vi "Send Current.vi"(8 "error in":errorcluster, 11 "6700C in":refnum<class "6700C.lvclass">) -> (0 "error out":errorcluster, 3 "6700C out":refnum<class "6700C.lvclass">)   [LabVIEW 2019, in "6700C.lvlib" / "6700C.lvclass"]
uses:
  Library/6700C.lvclass
  C:/Users/Public/Documents/Development/builds/Instruments/PowerSupply.lvlibp/Library/PowerSupply.lvclass
  Library/6700C.lvclass/6700C.ctl
  Accessors/Read Local Resource.vi
  Accessors/Write Local Resource.vi
  builds/Instruments/PowerSupply.lvlibp/Accessors/Read Active Channel.vi
  <instrlib>/Agilent N6700 Series/Agilent N6700 Series.lvlib
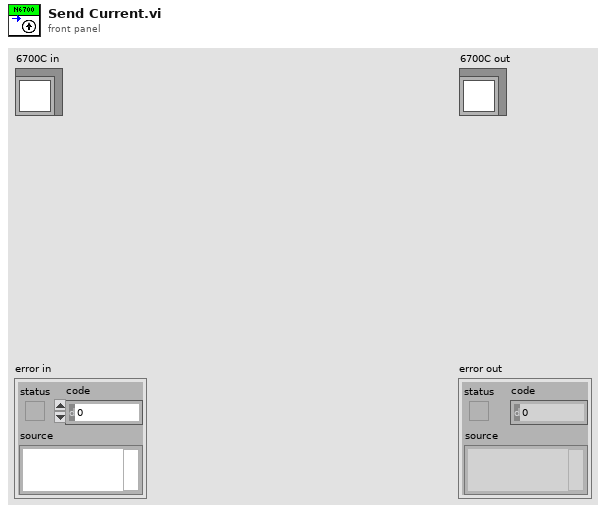
[diagram p1: front panel]
types:
  T1 = typedef "PowerSupply.lvlibp/PowerSupply.lvclass/OCP Mode.ctl" = enum16{"Shutdown", "Foldback"}
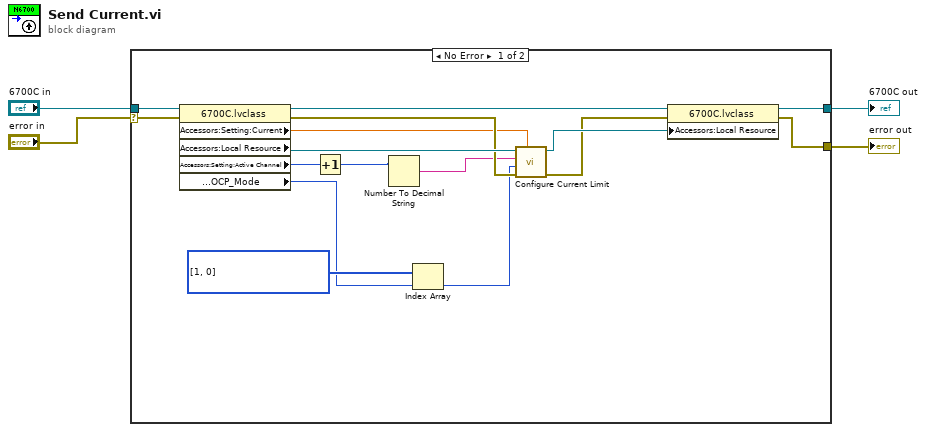
[diagram p0: block diagram]
diagram:
  n1 = case shown="No Error" "error in" {
    selector: "error in" -> [w12 w22]
    tunnel: [w14 w22] -> w4
    tunnel: [w15 w21] -> w3
    tunnel: "6700C in" -> [w20 w21]
    frame No Error {
      w8 = i32[] [1, 0] items=["Regulatory Limit", "Trip Limit"]
      n2 = property class="6700C.lvclass"(reference=w20, error in=w12) -> (reference out=w16:refnum<class "6700C.lvclass">, error out=w18:errorcluster, "Accessors:Setting:Current"=w11:dbl, "Accessors:Local Resource"=w19:refnum<visa-resource-name>, "Accessors:Setting:Active Channel"=w9:u32, "Accessors:Setting:Protection:OCP_Mode"=w7:T1)
      n3 = Increment(x=w9) -> (x+1=w5:u32)
      n4 = Number To Decimal String(number=w5) -> (decimal integer string=w10:string)  [unwired: 1 in]
      n5 = Index Array(array=w8, index=w7) -> (element=w6:i32)
      n6 = call <instrlib>:"Configure Current Limit.vi"("Limit (0.0 amps)"=w11, "error in (no error)"=w18, "Behavior (0: Regulatory Limit)"=w6, "Channel Name (1)"=w10, "VISA resource name"=w19) -> ("error out"=w13:errorcluster, "VISA resource name out"=w17:refnum<visa-resource-name>)  [unwired: 5 in]
      n7 = property class="6700C.lvclass"(reference=w16, error in=w13, "Accessors:Local Resource"=w17) -> (reference out=w15:refnum<class "6700C.lvclass">, error out=w14:errorcluster)
    }
    frame Error {
    }
  }
  "error out" <- w4
  "6700C out" <- w3
